vi "send command to camera.vi"(8 "error in (no error)":errorcluster, 11 "Autofocus in":refnum<class "Autofocus.lvclass">) -> (0 "error out":errorcluster, 3 "Autofocus out":refnum<class "Autofocus.lvclass">)   [LabVIEW 2012, in "Autofocus.lvclass"]
uses:
  Autofocus.lvclass
  <vilib>/Distrio/Murmex/StartMessage/run mode enum.ctl
  <vilib>/Distrio/Murmex/Murmex/update_cluster.ctl
  <vilib>/Distrio/Murmex/StartMessage/StartMessage.lvclass
  Autofocus.lvclass/Autofocus.ctl
  <vilib>/Distrio/Murmex/Murmex/Murmex.lvclass
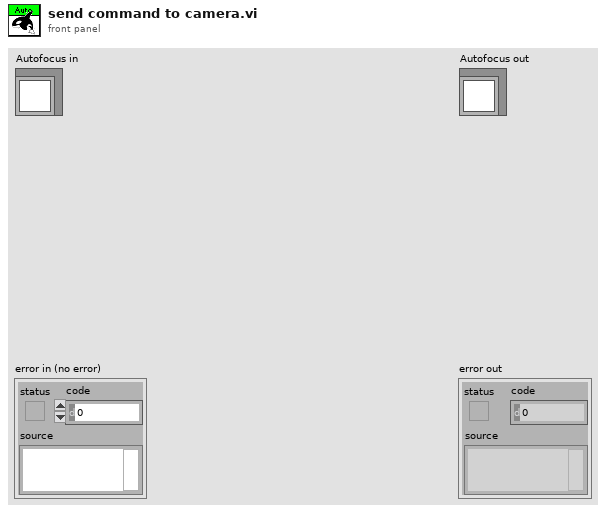
[diagram p1: front panel]
types:
  T1 = typedef "Murmex.lvlib/Murmex.lvclass/update_cluster.ctl" = cluster{"target ID":string, "key chains":string[], "values":variant[]}
  T2 = typedef "Murmex.lvlib/StartMessage.lvclass/run mode enum.ctl" = enum16{"infinite", "finite"}
  T3 = typedef "Autofocus.lvclass/image acquisition mode.ctl" = enum16{"Focus Stack", "Single Frame"}
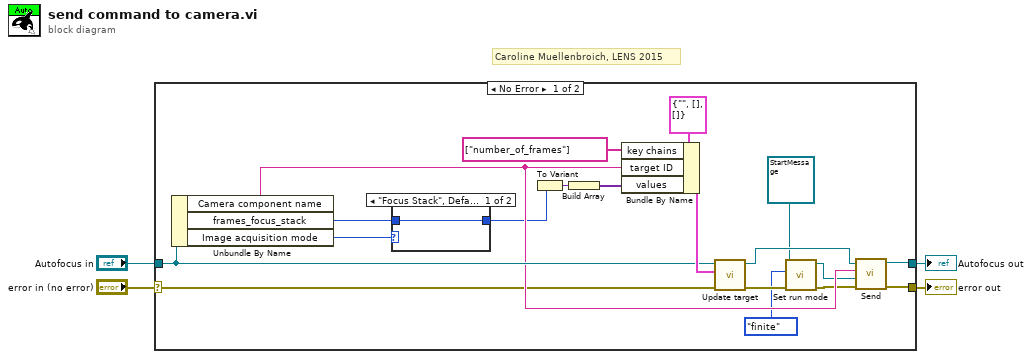
[diagram p0: block diagram]
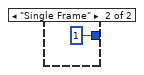
[diagram p2: hidden frame]
diagram:
  # "Caroline Muellenbroich, LENS 2015"
  n1 = case shown="No Error" "error in (no error)" {
    selector: "error in (no error)" -> [w14 w27]
    tunnel: [w17 w27] -> w3
    tunnel: [w16 w26] -> w1
    tunnel: "Autofocus in" -> [w18 w26]
    frame No Error {
      n2 = Unbundle By Name(w18) -> ("Camera component name"=w15:string, "frames_focus_stack"=w5:u16, "Image acquisition mode"=w7:T3)
      n3 = case shown="\"Focus Stack\", Default" w7 {
        tunnel: [w24 u16 1 ("frames_focus_stack")] -> w6
        tunnel: w5 -> [w24 _]
        frame "Focus Stack", Default {
        }
        frame "Single Frame" {
        }
      }
      n4 = To Variant(anything=w6) -> (Variant=w22:variant)
      n5 = Build Array(w22) -> (w21:variant[])
      n6 = Bundle By Name(cluster=T1 {"target ID"="", "key chains"=[], "values"=[]} ("update cluster"), "key chains"=string[] ["number_of_frames"], "target ID"=w15, "values"=w21) -> (w20:T1)
      n7 = call <vilib>:"Update target.vi"("error in (no error)"=w14, "update cluster"=w20, "MurmexBase in"=w18) -> ("error out"=w13:errorcluster, "MurmexBase out"=w11:refnum<class "Autofocus.lvclass">)  [unwired: 7 in]
      n8 = call <vilib>:"Set run mode.vi"("error in (no error)"=w13, "run mode"=run_mode_enum."finite", "StartMessage in"=refnum<class "StartMessage.lvclass"> refnum ("Distrio Murmex 1.5:StartMessage")) -> ("error out"=w12:errorcluster, "StartMessage out"=w10:refnum<class "StartMessage.lvclass">)  [unwired: 7 in]
      n9 = call <vilib>:"Send.vi"("error in (no error)"=w12, "Message"=w10, "recipient"=w15, "Murmex in"=w11) -> ("error out"=w17:errorcluster, "Murmex out"=w16:refnum<class "Autofocus.lvclass">)  [unwired: 6 in]
    }
    frame Error {
    }
  }
  "error out" <- w3
  "Autofocus out" <- w1
